vi "Kill Process.vi"(8 "error in (no error)":errorcluster, 10 "Process ID":string, 11 "Tamer in":refnum<class "Tamer.lvclass">) -> (0 "error out":errorcluster, 3 "Tamer out":refnum<class "Tamer.lvclass">)   [LabVIEW 2020, in "Tamer.lvlib" / "Tamer.lvclass"]
uses:
  Tamer.lvclass
  TALOS/TALOS_PPL.lvlibp/Support VIs/Global Memory.vi
  TALOS/TALOS_PPL.lvlibp/Classes/uService List/Get Queue.vi
  TALOS/TALOS_PPL.lvlibp/Interfaces/FPGA Interface/FPGA Interface.lvclass
  TALOS/TALOS_PPL.lvlibp
  TALOS/TALOS_PPL.lvlibp/Classes/uService List/uService List.lvclass
  TALOS/Actor Framework.lvlibp/1abvi3w/vi.lib/ActorFramework/Stop Msg/Stop Msg.lvclass
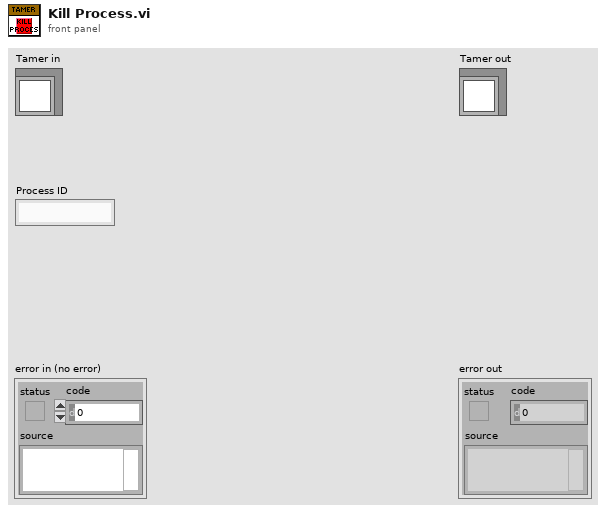
[diagram p1: front panel]
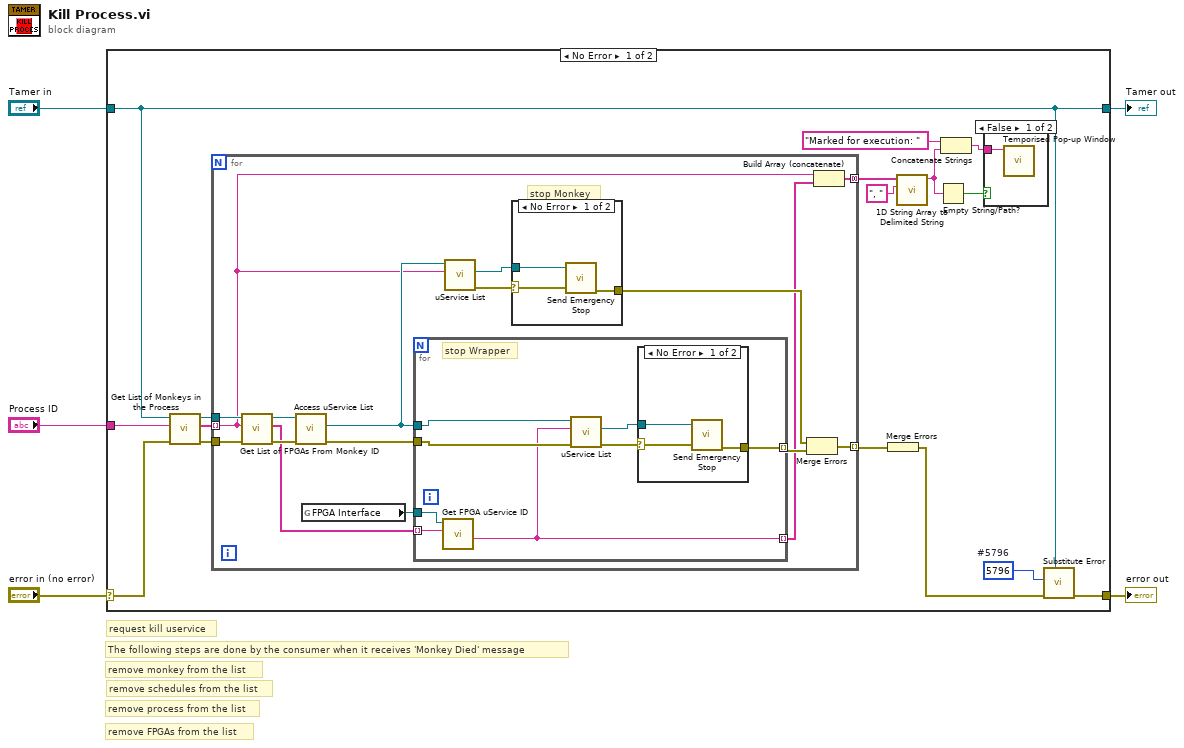
[diagram p0: block diagram]
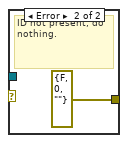
[diagram p3: hidden frame]
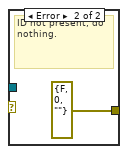
[diagram p4: hidden frame]
diagram:
  # "The following steps are done by the consumer when it receives 'Monkey Died' message"
  # "remove FPGAs from the list"
  # "remove process from the list"
  # "remove schedules from the list"
  # "remove monkey from the list"
  # "request kill uservice"
  n1 = case shown="No Error" "error in (no error)" {
    selector: "error in (no error)" -> [w18 w56]
    tunnel: [w14 w56] -> w4
    tunnel: [w12 w55] -> w2
    tunnel: "Tamer in" -> [w12 w55]
    tunnel: "Process ID" -> [w21 _]
    frame No Error {
      w13 = 5796  # #5796
      n2 = call-dynamic "Get List of Monkeys in the Process.vi"("error in (no error)"=w18, "Process ID"=w21, "Tamer in"=w12) -> ("error out"=w19:errorcluster, "List of Monkeys"=w17:string[], "Tamer out"=w20:refnum<class "Tamer.lvclass">)  [unwired: 5 in, 1 out]
      n3 = for {
        tunnel: w20 -> [w38]
        tunnel: w19 -> [w37]
        tunnel: w17 -> [w24] mode=indexing
        tunnel: [w26] -> w16 mode=indexing
        tunnel: [w23] -> w11 mode=concatenating
        # "stop Monkey"
        n4 = call-dynamic "Get List of FPGAs From Monkey ID.vi"("error in (no error)"=w37, "Monkey ID"=w24, "Tamer in"=w38) -> ("error out"=w34:errorcluster, "FPGA Names"=w33:string[], "Tamer out"=w35:refnum<class "Tamer.lvclass">)  [unwired: 5 in, 1 out]
        n5 = call-dynamic "Access uService List.vi"("error in (no error)"=w34, "Ancestor in"=w35) -> ("error out"=w32:errorcluster, "uService List out"=w29:refnum<class "uService List.lvclass">)  [unwired: 7 in, 1 out]
        n6 = global read "Global Memory.vi" "FPGA Interface"() -> (w36:refnum<class "FPGA Interface.lvclass">)
        n7 = for {
          tunnel: w33 -> [w49] mode=indexing
          tunnel: w36 -> [w50]
          tunnel: w29 -> [w46]
          tunnel: w32 -> [w45]
          tunnel: [w44] -> w28 mode=indexing
          tunnel: [w43] -> w25 mode=indexing
          # "stop Wrapper"
          n8 = call-dynamic "Get FPGA uService ID.vi"("FPGA Name"=w49, "FPGA Interface"=w50) -> ("uService ID"=w43:string)  [unwired: 5 in, 2 out]
          n9 = call-poly "uService List.vi"("error in (no error)"=w45, "ID"=w43, "uService List in"=w46) -> ("error out"=w47:errorcluster, "uService Queue"=w48:refnum<class "Message Enqueuer.lvclass">)  [unwired: 6 in, 1 out]
          n10 = case shown="No Error" w47 {
            selector: w47 -> [w51 _]
            tunnel: w48 -> [w53 _]
            tunnel: [w52 errorcluster {"status"=FALSE, "code"=0, "source"=""} ("error out")] -> w44
            frame No Error {
              n11 = call "Send Emergency Stop.vi"("error in (no error)"=w51, "Message Enqueuer"=w53) -> ("error out"=w52:errorcluster)  [unwired: 9 in]
            }
            frame Error {
              # "ID not present, do nothing."
            }
          }
        }
        n12 = call-poly "uService List.vi"("ID"=w24, "uService List in"=w29) -> ("error out"=w31:errorcluster, "uService Queue"=w30:refnum<class "Message Enqueuer.lvclass">)  [unwired: 7 in, 1 out]
        n13 = case shown="No Error" w31 {
          selector: w31 -> [w39 _]
          tunnel: w30 -> [w41 _]
          tunnel: [w40 errorcluster {"status"=FALSE, "code"=0, "source"=""} ("error out")] -> w27
          frame No Error {
            n14 = call "Send Emergency Stop.vi"("error in (no error)"=w39, "Message Enqueuer"=w41) -> ("error out"=w40:errorcluster)  [unwired: 9 in]
          }
          frame Error {
            # "ID not present, do nothing."
          }
        }
        n15 = Merge Errors(w27, w28) -> (w26:errorcluster)
        n16 = Build Array (concatenate)(w24, w25) -> (w23:string[])
      }
      n17 = Merge Errors(w16) -> (w15:errorcluster)
      n18 = call <vilib>:"1D String Array to Delimited String.vi"("delimiter"=", ", "string array"=w11) -> ("delimited string"=w7:string)  [unwired: 9 in]
      n19 = Empty String/Path?(string/path=w7) -> (empty?=w6:bool)
      n20 = Concatenate Strings("Marked for execution: ", w7) -> (w8:string)
      n21 = case shown="False" w6 {
        tunnel: w8 -> [w22 _]
        frame False {
          n22 = call "Temporised Pop-up Window.vi"("Text"=w22) -> ()  [unwired: 10 in, 1 out]
        }
        frame True {
        }
      }
      n23 = call "Substitute Error.vi"("LabVIEW Object"=w12, "error in (no error)"=w15, "Error Code"=w13) -> ("error out"=w14:errorcluster)  [unwired: 8 in]
    }
    frame Error {
    }
  }
  "error out" <- w4
  "Tamer out" <- w2
